vi "THCD_401_Main.vi"() -> ()   [LabVIEW 2019]
uses:
  THCD_400/thcd_controls/ctrl_sms_thcd.ctl
  THCD_401_Global.vi
panel:
  in  "reinit_PID":bool
  in  "flow_ch2_min":dbl
  in  "flow_ch2_max":dbl=50.0
  out "status_auto_ctrl_ch2":u32(colorbox) caption="Control Status"
  out "sp_ch2_org":dbl=100.0 min=0.1 max=10000.0 format="%#_5f"
  in  "enable_auto_ctrl_ch2":bool caption="Automation"
  out "sp_ch1_org":dbl=100.0 min=0.1 max=10000.0 format="%#_5f"
  out "msg_cont_ch2":string caption="Msg"
  out "status_auto_ctrl":u32(colorbox) caption="Control Status"
  in  "P_mag_set":dbl=0.5 caption="Set Point" format="%.2f"
  in  "enable_auto_ctrl":bool caption="Automation"
  out "P_mag_psi":dbl=1.1 format="%.2f"
  out "P_mag_Torr":dbl caption="Magnet Pressure" format="%_4f"
  out "current_sp_ch2":dbl caption="Current S.P."
  out "status_ch2":bool caption="Status"
  in  "set_mode_ch2":enum16{"AUTO", "OPEN", "CLOSE"}(ring) caption="Change mode to"
  in  "set_sp_ch2":dbl=100.0 caption="Change S.P. to" min=0.0 max=1000.0 step=1.0 format="%#_5f"
  out "msg_cont":string caption="Msg"
  in  "set_mode_ch1":enum16{"AUTO", "OPEN", "CLOSE"}(ring) caption="Change mode to"
  out "mode_ch2":string
  out "mode_ch1":string
  out "Chart":waveform(dbl)[](graph)=[{"t0"=timestamp(3748719860.656619 s since 1904-01-01), "dt"=1.0, "Y"=[3.092]}, {"t0"=timestamp(3748719860.656619 s since 1904-01-01), "dt"=1.0, "Y"=[6.266]}, {"t0"=timestamp(3748719860.656619 s since 1904-01-01), "dt"=1.0, "Y"=[3.191]}]
  out "status_read":bool caption="Status"
  in  "Port":u16=101
  in  "Address":string="192.168.24.186"
  out "current_sp_ch1":dbl caption="Current S.P."
  out "status_log":bool caption="Status"
  in  "Logging":bool=TRUE
  out "Last Updated":timestamp format="%<%Y-%m-%d %H:%M:%S>T"
  out "status_ch1":bool caption="Status"
  in  "set_sp_ch1":dbl caption="Change S.P. to" min=0.0 max=1000.0 step=1.0 format="%#_5f"
  in  "wait_sec":u32=1 caption="Interval (s)"
  in  "read":bool
  out "FM1":dbl caption="L/m" format="%.3f"
  out "FC2":dbl caption="L/m" format="%.3f"
  out "FC1":dbl caption="L/m" format="%.3f"
  in  "Init Devices":bool
  in  "stop":bool
  # "THCD-401 :  Mass Flow Control & Monitor"
  # "The pressure used for the automation is measured with MaxiGauge.  It has an offset from that on QT HMI."
  # "Monitoring"
  # "Mode"
  # "S.P."
  # "Torr ~"
  # "psig"
  # "psig"
  # "Flow Control:  Magnet Return (FC1)"
  # "Flow Control:  Separator Return (FC2)"
  # "Flow Range:"
  # "-"
  # "L/m"
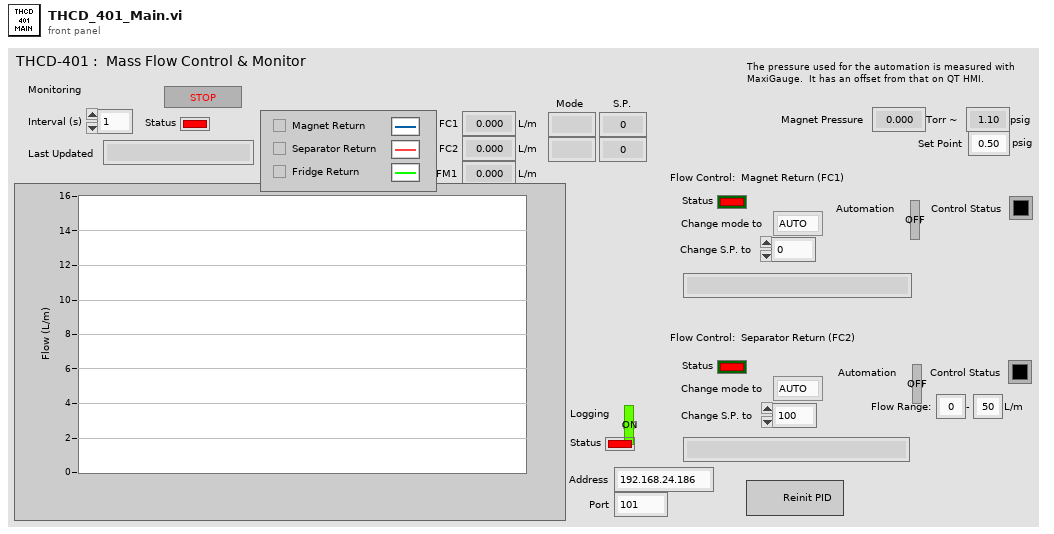
[diagram p1: front panel]
types:
  T1 = typedef "ctrl_sms_thcd.ctl" = enum16{"idle", "init", "exit", "read", "enable_auto_ctrl_ch1", "enable_auto_ctrl_ch2", "open", "close", "mode_ch1", "set", "open_ch2", "close_ch2", "mode_ch2", "set_ch2", "getstat"}
  T2 = enum8{"Enabled", "Disabled", "Disabled and Grayed Out"}
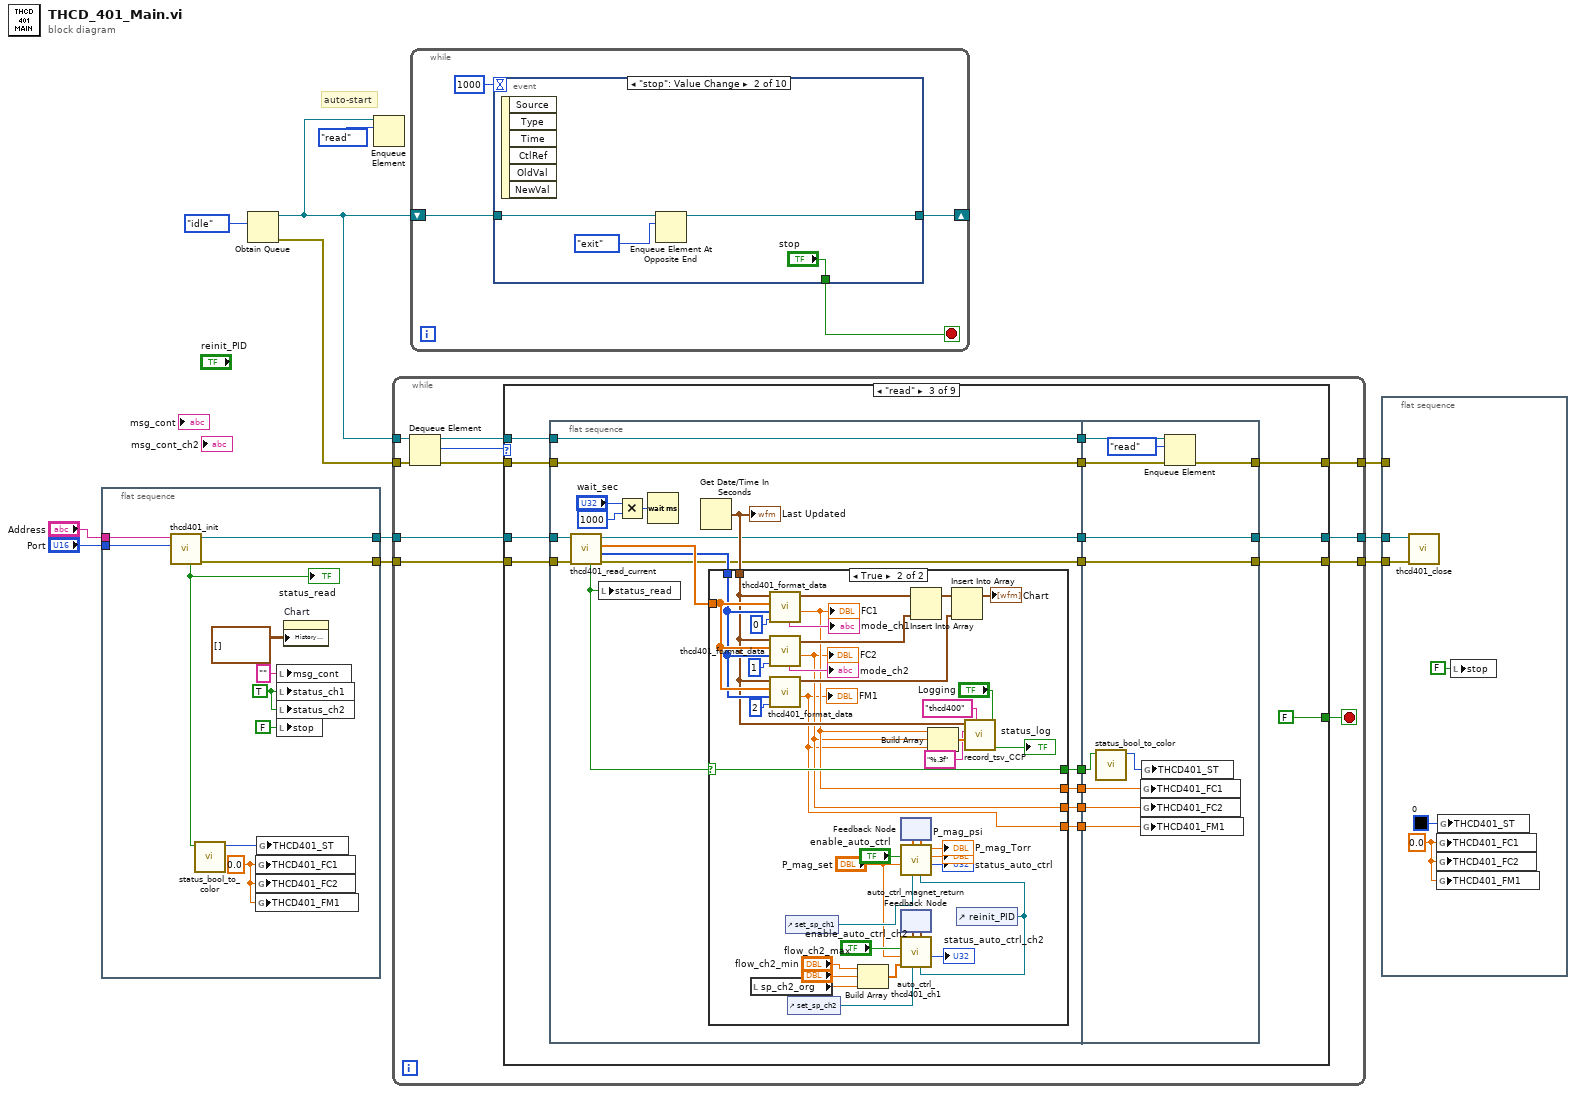
[diagram p0: block diagram]
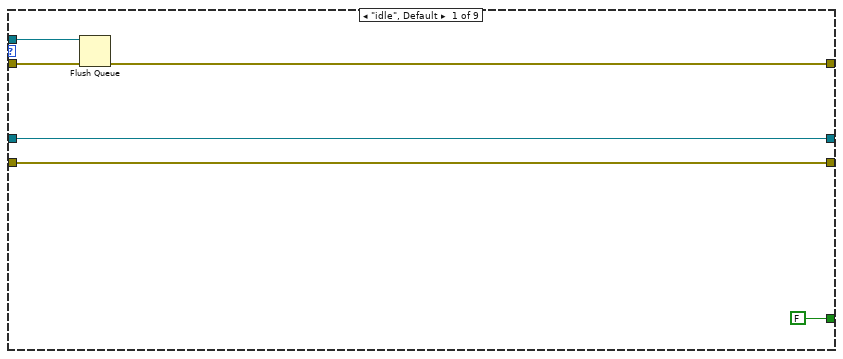
[diagram p2: hidden frame]
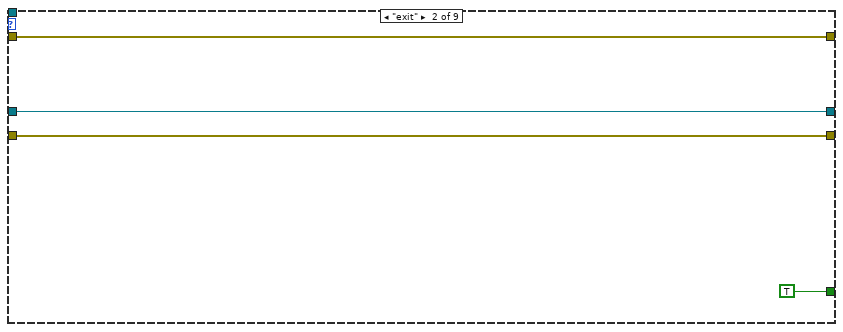
[diagram p3: hidden frame]
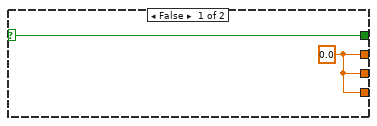
[diagram p4: hidden frame]
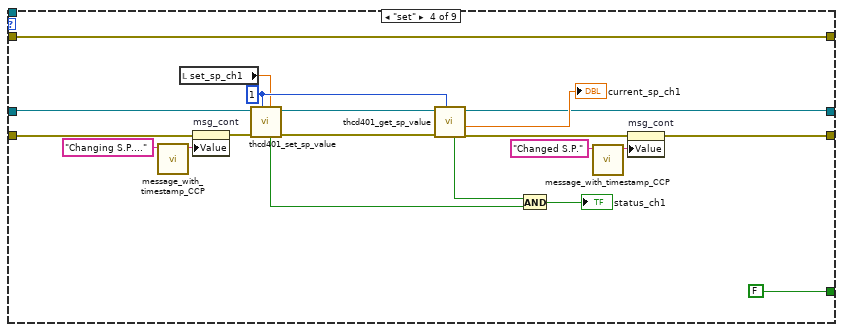
[diagram p5: hidden frame]
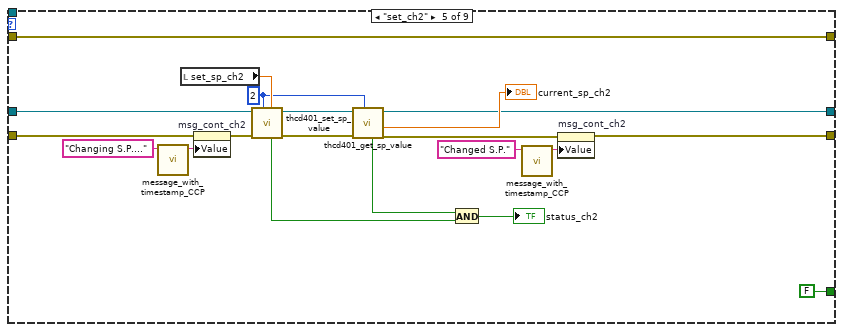
[diagram p6: hidden frame]
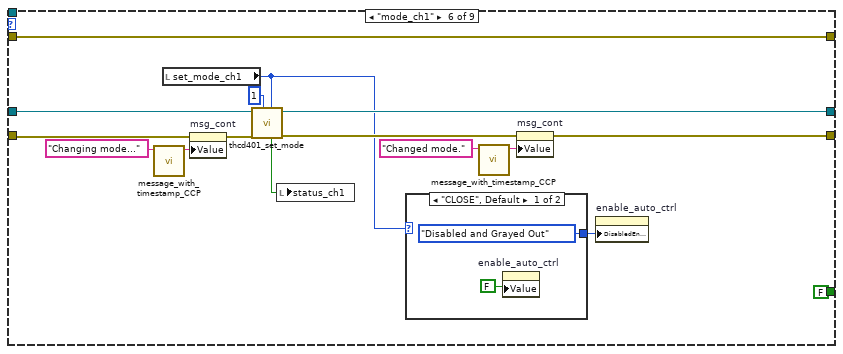
[diagram p7: hidden frame]
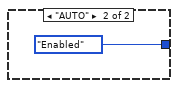
[diagram p8: hidden frame]
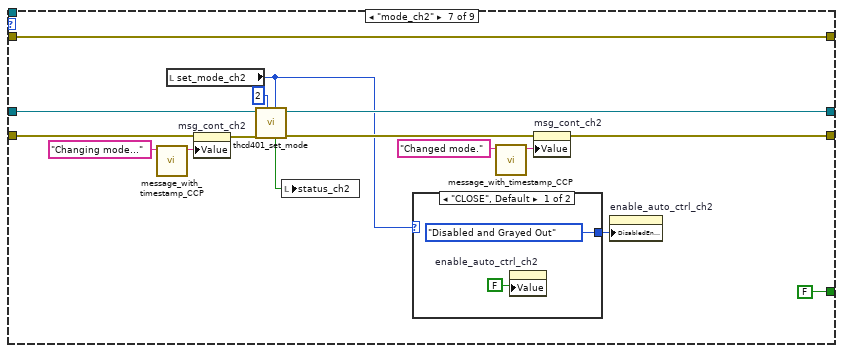
[diagram p9: hidden frame]
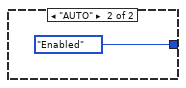
[diagram p10: hidden frame]
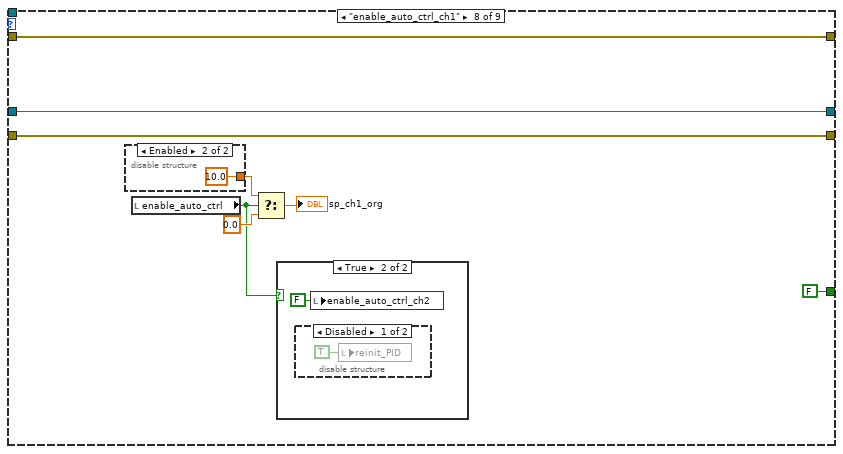
[diagram p11: hidden frame]
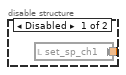
[diagram p12: hidden frame]
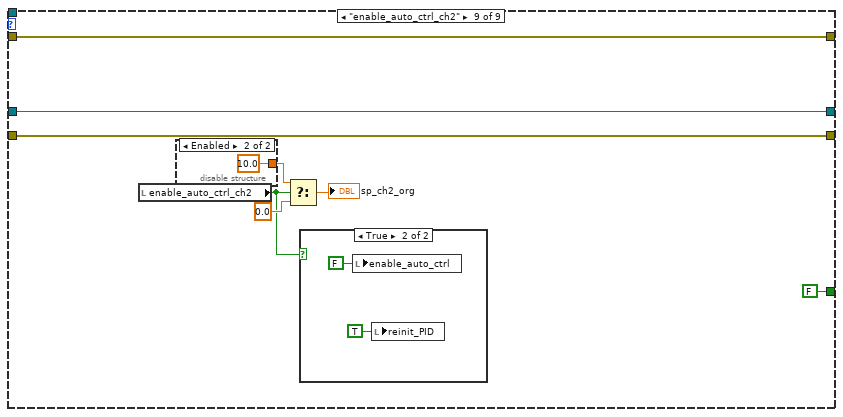
[diagram p15: hidden frame]
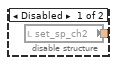
[diagram p16: hidden frame]
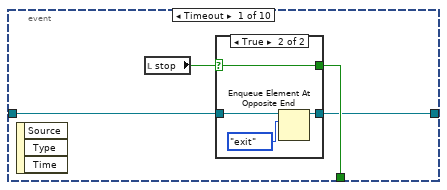
[diagram p18: hidden frame]
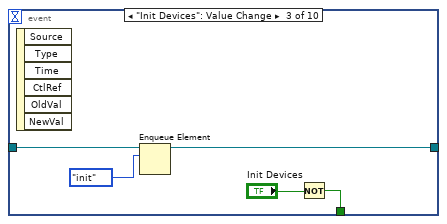
[diagram p20: hidden frame]
diagram:
  # "auto-start"
  n1 = flat-sequence {
    tunnel: "Address" -> [w22]
    tunnel: "Port" -> [w21]
    tunnel: [w20] -> w4
    tunnel: [w19] -> w1
    frame #0 {
      w15 = 0.0 ("THCD401_FC1")
      w16 = TRUE ("status_ch1")
      n2 = call "thcd401_init.vi"("port"=w21, "address"=w22) -> ("error out"=w19:errorcluster, "conn_id"=w20:refnum<k5>, "status"=w13:bool)  [unwired: 7 in]
      "status_read" <- w13
      n3 = call "status_bool_to_color.vi"("status_bool_1"=w13) -> ("status_color"=w14:u32)  [unwired: 10 in]
      n4 = global write "THCD_401_Global.vi" "THCD401_FC1"(w15) -> ()
      n5 = global write "THCD_401_Global.vi" "THCD401_FC2"(w15) -> ()
      n6 = global write "THCD_401_Global.vi" "THCD401_FM1"(w15) -> ()
      n7 = global write "THCD_401_Global.vi" "THCD401_ST"(w14) -> ()
      n8 = local write "msg_cont"("" ("msg_ch1")) -> ()
      n9 = local write "status_ch1"(w16) -> ()
      n10 = local write "status_ch2"(w16) -> ()
      n11 = local write "stop"(FALSE ("stop")) -> ()
      n12 = property on="Chart" class="WFChart (strict)"("History Data"=waveform(dbl)[][] []) -> ()  [unwired: 2 in, 2 out]
    }
  }
  n13 = Obtain Queue(element data type=ctrl_sms_thcd."idle" ("Enum")) -> (queue out=w8:refnum<queue>, error out=w10:errorcluster)  [unwired: 4 in, 1 out]
  n14 = Enqueue Element(queue=w8, element=ctrl_sms_thcd."read") -> ()  [unwired: 2 in, 3 out]
  n15 = while {
    tunnel: w10 -> [w31]
    tunnel: [w28] -> w7
    tunnel: w8 -> [w32]
    tunnel: w4 -> [w26]
    tunnel: [w25] -> w3
    tunnel: [w23] -> w2
    tunnel: w1 -> [w24]
    stop <- w33 stop-if-true
    n16 = Dequeue Element(queue=w32, error in (no error)=w31) -> (queue out=w27:refnum<queue>, element=w30:T1, error out=w29:errorcluster)  [unwired: 1 in, 1 out]
    n17 = case shown="\"read\"" w30 {
      tunnel: w27 -> [w38 _ w49 _ _ _ _ _ _]
      tunnel: [FALSE TRUE FALSE FALSE FALSE FALSE FALSE FALSE FALSE] -> w33
      tunnel: w29 -> [w37 w42 w51 w148 w169 w178 w204 w215 w227]
      tunnel: [w36 w42 w52 w148 w169 w178 w204 w215 w227] -> w28
      tunnel: w26 -> [w35 w41 w58 w147 w167 w182 w200 w214 w226]
      tunnel: [w35 w41 w56 w143 w158 w179 w198 w214 w226] -> w25
      tunnel: w24 -> [w34 w40 w57 w141 w166 w181 w199 w212 w225]
      tunnel: [w34 w40 w55 w138 w157 w180 w197 w212 w225] -> w23
      frame "idle", Default {
        n18 = Flush Queue(queue=w38, error in (no error)=w37) -> (error out=w36:errorcluster)  [unwired: 2 out]
      }
      frame "exit" {
      }
      frame "read" {
        n19 = flat-sequence {
          tunnel: w58 -> [w73]
          tunnel: w57 -> [w72]
          tunnel: [w68] -> w54
          tunnel: [w67] -> w53
          tunnel: w51 -> [w65]
          tunnel: [w65] -> w50
          tunnel: w49 -> [w64]
          tunnel: [w64] -> w48
          tunnel: [w63] -> w47
          tunnel: [w62] -> w46
          tunnel: [w61] -> w45
          tunnel: [w60] -> w44
          tunnel: [w128] -> w55
          tunnel: [w129] -> w56
          tunnel: w54 -> [w129]
          tunnel: w53 -> [w128]
          tunnel: [w126] -> w52
          tunnel: w50 -> [w125]
          tunnel: w48 -> [w124]
          tunnel: w47 -> [w123]
          tunnel: w46 -> [w121]
          tunnel: w45 -> [w120]
          tunnel: w44 -> [w119]
          frame #0 {
            n20 = call "thcd401_read_current.vi"("error in"=w72, "conn_id_in"=w73) -> ("error out"=w67:errorcluster, "mode_array"=w69:i32[], "value_array"=w70:dbl[], "conn_id_out"=w68:refnum<k5>, "status"=w66:bool)  [unwired: 5 in]
            n21 = local write "status_read"(w66) -> ()
            n22 = Multiply(x="wait_sec", y=u32 1000) -> (x*y=w76:u32)
            n23 = Wait (ms)(milliseconds to wait=w76) -> ()  [unwired: 1 out]
            n24 = Get Date/Time In Seconds() -> (seconds since 1Jan1904=w71:timestamp)
            "Last Updated" <- w71
            n25 = case shown="True" w66 {
              selector: w66 -> [w78 w82]
              tunnel: w71 -> [_ w102]
              tunnel: w70 -> [_ w115]
              tunnel: w69 -> [_ w114]
              tunnel: [w78 w82] -> w63
              tunnel: [w77 w81] -> w62
              tunnel: [w77 w80] -> w61
              tunnel: [w77 w79] -> w60
              frame False {
                w77 = 0.0 ("value")
              }
              frame True {
                n26 = local read "sp_ch2_org"() -> (w87:dbl)
                n27 = call "thcd401_format_data.vi"("index"=0, "mode_array"=w114, "value_array"=w115, "time"=w102) -> ("value"=w81:dbl, "waveform_array"=w113:waveform(dbl)[], "mode_str"=→"mode_ch1":string)  [unwired: 4 in, 1 out]
                "FC1" <- w81
                n28 = call "thcd401_format_data.vi"("index"=1, "mode_array"=w114, "value_array"=w115, "time"=w102) -> ("value"=w80:dbl, "waveform_array"=w112:waveform(dbl)[], "mode_str"=→"mode_ch2":string)  [unwired: 4 in, 1 out]
                "FC2" <- w80
                n29 = call "thcd401_format_data.vi"("index"=2, "mode_array"=w114, "value_array"=w115, "time"=w102) -> ("value"=w79:dbl, "waveform_array"=w110:waveform(dbl)[])  [unwired: 4 in, 2 out]
                "FM1" <- w79
                n30 = control-ref of="set_sp_ch1"() -> (w98:refnum<vi>)
                n31 = control-ref of="set_sp_ch2"() -> (w84:refnum<vi>)
                n32 = Build Array("flow_ch2_min", "flow_ch2_max", w87) -> (w86:dbl[])
                n33 = feedback #1() -> (w96:dbl[])  [unwired: 1 in]
                n34 = feedback #2() -> (w93:timestamp)  [unwired: 1 in]
                n35 = Insert Into Array(array=w113, new element=w112) -> (w111:waveform(dbl)[])  [unwired: 1 in]
                n36 = Build Array(w81, w80, w79) -> (w103:dbl[])
                n37 = Insert Into Array(array=w111, new element=w110) -> (→"Chart":waveform(dbl)[])  [unwired: 1 in]
                n38 = control-ref of="reinit_PID"() -> (w85:refnum<vi>)
                n39 = call "auto_ctrl_magnet_return.vi"("ref_reinit"=w85, "ref_sp_ch1"=w98, "array_value_in"=w96, "P_set"="P_mag_set", "enable_auto_ctrl"="enable_auto_ctrl") -> ("status"=→"status_auto_ctrl":u32, "P_psi"=→"P_mag_psi":dbl, "P_Torr"=→"P_mag_Torr":dbl, "array_value_out"=w97:dbl[])  [unwired: 2 in, 1 out]
                n40 = feedback-in #1(w97) -> ()
                n41 = call "auto_ctrl_thcd401_ch1.vi"("ref_reinit"=w85, "ref_sp_ch1"=w84, "time_last_ctrl_in"=w93, "flow_params"=w86, "P_set"="P_mag_set", "enable_auto_ctrl"="enable_auto_ctrl_ch2") -> ("status"=→"status_auto_ctrl_ch2":u32, "time_last_ctrl_out"=w94:timestamp)  [unwired: 1 in, 3 out]
                n42 = feedback-in #2(w94) -> ()
                n43 = call "record_tsv_CCP.vi"("logging_on"="Logging", "folder_name"="thcd400", "value_array"=w103, "format"="%.3f", "time"=w102) -> ("status"=→"status_log":bool)  [unwired: 5 in, 1 out]
              }
            }
          }
          frame #1 {
            n44 = call "status_bool_to_color.vi"("status_bool_1"=w123) -> ("status_color"=w122:u32)  [unwired: 10 in]
            n45 = global write "THCD_401_Global.vi" "THCD401_FC1"(w121) -> ()
            n46 = global write "THCD_401_Global.vi" "THCD401_FC2"(w120) -> ()
            n47 = global write "THCD_401_Global.vi" "THCD401_FM1"(w119) -> ()
            n48 = global write "THCD_401_Global.vi" "THCD401_ST"(w122) -> ()
            n49 = Enqueue Element(queue=w124, element=ctrl_sms_thcd."read", error in (no error)=w125) -> (error out=w126:errorcluster)  [unwired: 1 in, 2 out]
          }
        }
      }
      frame "set" {
        w146 = u8 1 ("channel")
        n50 = call "message_with_timestamp_CCP.vi"("message_in"="Changing S.P...." ("msg_ch1")) -> ("message_out"=w133:string)  [unwired: 10 in]
        n51 = local read "set_sp_ch1"() -> (w134:dbl)
        n52 = property on="msg_cont" class="Str"(error in=w141, "Value"=w133) -> (error out=w140:errorcluster)  [unwired: 1 in, 1 out]
        n53 = call "thcd401_set_sp_value.vi"("value"=w134, "channel"=w146, "error in"=w140, "conn_id_in"=w147) -> ("error out"=w142:errorcluster, "conn_id_out"=w145:refnum<k5>, "status"=w135:bool)  [unwired: 5 in]
        n54 = call "thcd401_get_sp_value.vi"("channel"=w146, "error in"=w142, "conn_id_in"=w145) -> ("error out"=w139:errorcluster, "value"=→"current_sp_ch1":dbl, "conn_id_out"=w143:refnum<k5>, "status"=w136:bool)  [unwired: 4 in, 1 out]
        n55 = And(x=w136, y=w135) -> (x .and. y?=→"status_ch1":bool)
        n56 = call "message_with_timestamp_CCP.vi"("message_in"="Changed S.P." ("msg_ch1")) -> ("message_out"=w131:string)  [unwired: 10 in]
        n57 = property on="msg_cont" class="Str"(error in=w139, "Value"=w131) -> (error out=w138:errorcluster)  [unwired: 1 in, 1 out]
      }
      frame "set_ch2" {
        w155 = u8 2 ("channel")
        n58 = call "message_with_timestamp_CCP.vi"("message_in"="Changing S.P...." ("msg_ch1")) -> ("message_out"=w153:string)  [unwired: 10 in]
        n59 = local read "set_sp_ch2"() -> (w165:dbl)
        n60 = property on="msg_cont_ch2" class="Str"(error in=w166, "Value"=w153) -> (error out=w168:errorcluster)  [unwired: 1 in, 1 out]
        n61 = call "thcd401_set_sp_value.vi"("value"=w165, "channel"=w155, "error in"=w168, "conn_id_in"=w167) -> ("error out"=w159:errorcluster, "conn_id_out"=w160:refnum<k5>, "status"=w156:bool)  [unwired: 5 in]
        n62 = call "thcd401_get_sp_value.vi"("channel"=w155, "error in"=w159, "conn_id_in"=w160) -> ("error out"=w163:errorcluster, "value"=→"current_sp_ch2":dbl, "conn_id_out"=w158:refnum<k5>, "status"=w161:bool)  [unwired: 4 in, 1 out]
        n63 = And(x=w161, y=w156) -> (x .and. y?=→"status_ch2":bool)
        n64 = call "message_with_timestamp_CCP.vi"("message_in"="Changed S.P." ("msg_ch1")) -> ("message_out"=w151:string)  [unwired: 10 in]
        n65 = property on="msg_cont_ch2" class="Str"(error in=w163, "Value"=w151) -> (error out=w157:errorcluster)  [unwired: 1 in, 1 out]
      }
      frame "mode_ch1" {
        n66 = call "message_with_timestamp_CCP.vi"("message_in"="Changing mode..." ("msg_ch1")) -> ("message_out"=w175:string)  [unwired: 10 in]
        n67 = local read "set_mode_ch1"() -> (w171:enum16{"AUTO", "OPEN", "CLOSE"})
        n68 = property on="msg_cont" class="Str"(error in=w181, "Value"=w175) -> (error out=w184:errorcluster)  [unwired: 1 in, 1 out]
        n69 = call "thcd401_set_mode.vi"("mode"=w171, "channel"=u8 1, "error in"=w184, "conn_id_in"=w182) -> ("error out"=w183:errorcluster, "conn_id_out"=w179:refnum<k5>, "status"=w176:bool)  [unwired: 5 in]
        n70 = local write "status_ch1"(w176) -> ()
        n71 = case shown="\"CLOSE\", Default" w171 {
          tunnel: [T2."Disabled and Grayed Out" ("Disabled") T2."Enabled" ("Disabled")] -> w170
          frame "CLOSE", Default {
            n72 = property on="enable_auto_ctrl" class="Bool (strict)"("Value"=FALSE ("enable_auto_ctrl")) -> ()  [unwired: 2 in, 2 out]
          }
          frame "AUTO" {
          }
        }
        n73 = call "message_with_timestamp_CCP.vi"("message_in"="Changed mode." ("msg_ch1")) -> ("message_out"=w173:string)  [unwired: 10 in]
        n74 = property on="msg_cont" class="Str"(error in=w183, "Value"=w173) -> (error out=w180:errorcluster)  [unwired: 1 in, 1 out]
        n75 = property on="enable_auto_ctrl" class="Bool (strict)"("DisabledEnum"=w170) -> ()  [unwired: 2 in, 2 out]
      }
      frame "mode_ch2" {
        n76 = call "message_with_timestamp_CCP.vi"("message_in"="Changing mode..." ("msg_ch1")) -> ("message_out"=w194:string)  [unwired: 10 in]
        n77 = local read "set_mode_ch2"() -> (w190:enum16{"AUTO", "OPEN", "CLOSE"})
        n78 = property on="msg_cont_ch2" class="Str"(error in=w199, "Value"=w194) -> (error out=w202:errorcluster)  [unwired: 1 in, 1 out]
        n79 = call "thcd401_set_mode.vi"("mode"=w190, "channel"=u8 2, "error in"=w202, "conn_id_in"=w200) -> ("error out"=w201:errorcluster, "conn_id_out"=w198:refnum<k5>, "status"=w195:bool)  [unwired: 5 in]
        n80 = local write "status_ch2"(w195) -> ()
        n81 = case shown="\"CLOSE\", Default" w190 {
          tunnel: [T2."Disabled and Grayed Out" ("Disabled") T2."Enabled" ("Disabled")] -> w189
          frame "CLOSE", Default {
            n82 = property on="enable_auto_ctrl_ch2" class="Bool (strict)"("Value"=FALSE ("enable_auto_ctrl")) -> ()  [unwired: 2 in, 2 out]
          }
          frame "AUTO" {
          }
        }
        n83 = call "message_with_timestamp_CCP.vi"("message_in"="Changed mode." ("msg_ch1")) -> ("message_out"=w192:string)  [unwired: 10 in]
        n84 = property on="msg_cont_ch2" class="Str"(error in=w201, "Value"=w192) -> (error out=w197:errorcluster)  [unwired: 1 in, 1 out]
        n85 = property on="enable_auto_ctrl_ch2" class="Bool (strict)"("DisabledEnum"=w189) -> ()  [unwired: 2 in, 2 out]
      }
      frame "enable_auto_ctrl_ch1" {
        n86 = disable-structure shown="Enabled" {
          disable-tunnel: [w216 10.0 ("set_sp_ch1")] -> w210
          frame Disabled {
            n87 = local read "set_sp_ch1"() -> (w216:dbl)
          }
          frame Enabled {
          }
        }
        n88 = local read "enable_auto_ctrl"() -> (w208:bool)
        n89 = Select(t=w210, s=w208, f=0.0 ("sp_ch1_org")) -> (s? t:f=→"sp_ch1_org":dbl)
        n90 = case shown="True" w208 {
          frame False {
          }
          frame True {
            n91 = disable-structure shown="Disabled" {
              frame Disabled {
                n92 = local write "reinit_PID"(TRUE ("reinit_PID")) -> ()
              }
              frame Enabled {
              }
            }
            n93 = local write "enable_auto_ctrl_ch2"(FALSE ("enable_auto_ctrl_ch2")) -> ()
          }
        }
      }
      frame "enable_auto_ctrl_ch2" {
        n94 = local read "enable_auto_ctrl_ch2"() -> (w220:bool)
        n95 = disable-structure shown="Enabled" {
          disable-tunnel: [w228 10.0 ("set_sp_ch2")] -> w224
          frame Disabled {
            n96 = local read "set_sp_ch2"() -> (w228:dbl)
          }
          frame Enabled {
          }
        }
        n97 = Select(t=w224, s=w220, f=0.0) -> (s? t:f=→"sp_ch2_org":dbl)
        n98 = case shown="True" w220 {
          frame False {
          }
          frame True {
            n99 = local write "enable_auto_ctrl"(FALSE ("enable_auto_ctrl")) -> ()
            n100 = local write "reinit_PID"(TRUE ("reinit_PID")) -> ()
          }
        }
      }
    }
  }
  n101 = while {
    shift-right: [w234] -> _
    shift-left: w8 -> [w235]
    stop <- w233 stop-if-true
    n102 = event shown="[1] \"stop\": Value Change" {
      selector: _ -> [_ _ _ _ _ _ _ _ _ _]
      dyn-events: _ -> [_ _ _ _ _ _ _ _ _ _]
      timeout: 1000 -> [_ _ _ _ _ _ _ _ _ _]
      tunnel: w235 -> [w238 w249 w254 w257 w261 w265 w269 w273 w278 w282]
      tunnel: [w237 w248 w253 w256 w260 w264 w268 w272 w277 w281] -> w234
      tunnel: [w239 "stop" w250 FALSE ("Exit") FALSE ("Exit") FALSE ("Exit") FALSE ("Exit") w274 FALSE ("Exit") FALSE ("Exit")] -> w233
      event Timeout {
        n103 = event-data() -> ()  [unwired: 1 in, 3 out]
        n104 = local read "stop"() -> (w236:bool)
        n105 = case shown="True" w236 {
          selector: w236 -> [w241 w245]
          tunnel: [w241 w245] -> w239
          tunnel: w238 -> [w240 w242]
          tunnel: [w240 w243] -> w237
          frame False {
          }
          frame True {
            n106 = Enqueue Element At Opposite End(queue=w242, element=ctrl_sms_thcd."exit" ("Enum")) -> (queue out=w243:refnum<queue>)  [unwired: 2 in, 2 out]
          }
        }
      }
      event "stop": Value Change {
        n107 = event-data() -> ()  [unwired: 1 in, 6 out]
        n108 = Enqueue Element At Opposite End(queue=w249, element=ctrl_sms_thcd."exit" ("Enum")) -> (queue out=w248:refnum<queue>)  [unwired: 2 in, 2 out]
      }
      event "Init Devices": Value Change {
        n109 = event-data() -> ()  [unwired: 1 in, 6 out]
        n110 = Enqueue Element(queue=w254, element=ctrl_sms_thcd."init") -> (queue out=w253:refnum<queue>)  [unwired: 2 in, 2 out]
        n111 = Not(x="Init Devices") -> (.not. x?=w250:bool)
      }
      event "set_sp_ch1": Value Change {
        n112 = event-data() -> ()  [unwired: 1 in, 6 out]
        n113 = Enqueue Element(queue=w257, element=ctrl_sms_thcd."set" ("Enum")) -> (queue out=w256:refnum<queue>)  [unwired: 2 in, 2 out]
      }
      event "set_sp_ch2": Value Change {
        n114 = event-data() -> ()  [unwired: 1 in, 6 out]
        n115 = Enqueue Element(queue=w261, element=ctrl_sms_thcd."set_ch2" ("Enum")) -> (queue out=w260:refnum<queue>)  [unwired: 2 in, 2 out]
      }
      event "set_mode_ch1": Value Change {
        n116 = event-data() -> ()  [unwired: 1 in, 6 out]
        n117 = Enqueue Element(queue=w265, element=ctrl_sms_thcd."mode_ch1" ("Enum")) -> (queue out=w264:refnum<queue>)  [unwired: 2 in, 2 out]
      }
      event "set_mode_ch2": Value Change {
        n118 = event-data() -> ()  [unwired: 1 in, 6 out]
        n119 = Enqueue Element(queue=w269, element=ctrl_sms_thcd."mode_ch2" ("Enum")) -> (queue out=w268:refnum<queue>)  [unwired: 2 in, 2 out]
      }
      event "read": Value Change {
        n120 = event-data() -> ()  [unwired: 1 in, 6 out]
        n121 = Enqueue Element(queue=w273, element=ctrl_sms_thcd."read" ("Enum")) -> (queue out=w272:refnum<queue>)  [unwired: 2 in, 2 out]
        n122 = Not(x="read") -> (.not. x?=w274:bool)
      }
      event "enable_auto_ctrl": Value Change {
        n123 = event-data() -> ()  [unwired: 1 in, 6 out]
        n124 = Enqueue Element(queue=w278, element=ctrl_sms_thcd."enable_auto_ctrl_ch1" ("Enum")) -> (queue out=w277:refnum<queue>)  [unwired: 2 in, 2 out]
      }
      event "enable_auto_ctrl_ch2": Value Change {
        n125 = event-data() -> ()  [unwired: 1 in, 6 out]
        n126 = Enqueue Element(queue=w282, element=ctrl_sms_thcd."enable_auto_ctrl_ch2" ("Enum")) -> (queue out=w281:refnum<queue>)  [unwired: 2 in, 2 out]
      }
    }
  }
  n127 = flat-sequence {
    tunnel: w7 -> [_]
    tunnel: w3 -> [w288]
    tunnel: w2 -> [w287]
    frame #0 {
      w285 = 0.0 ("THCD401_FC1")
      n128 = call "thcd401_close.vi"("error in"=w287, "conn_id"=w288) -> ()  [unwired: 8 in, 2 out]
      n129 = global write "THCD_401_Global.vi" "THCD401_FC1"(w285) -> ()
      n130 = global write "THCD_401_Global.vi" "THCD401_FC2"(w285) -> ()
      n131 = global write "THCD_401_Global.vi" "THCD401_FM1"(w285) -> ()
      n132 = global write "THCD_401_Global.vi" "THCD401_ST"(u32 0 ("THCD401_ST")) -> ()
      n133 = local write "stop"(FALSE ("stop")) -> ()
    }
  }
